vi "Close.vi"(8 "error in (no error)":errorcluster, 11 "SSI PR Settings In":T1={"VISA resource name"="", "Simulated?"=TRUE}) -> (0 "error out":errorcluster, 3 "SSI PR Settings Out":T1={"VISA resource name"="", "Simulated?"=TRUE})   [LabVIEW 2018]
uses:
  SSI PR Settings Cluster.ctl
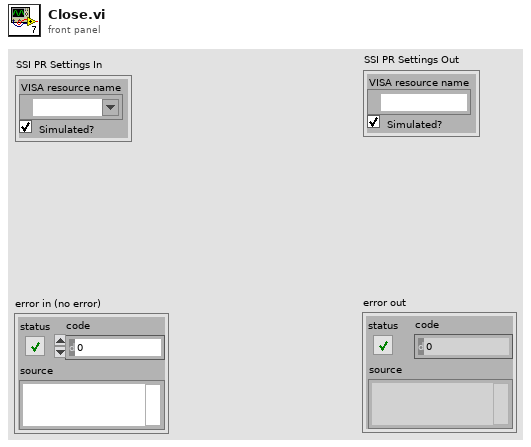
[diagram p1: front panel]
types:
  T1 = typedef "SSI PR Settings Cluster.ctl" = cluster{"VISA resource name":refnum<visa-resource-name>, "Simulated?":bool}
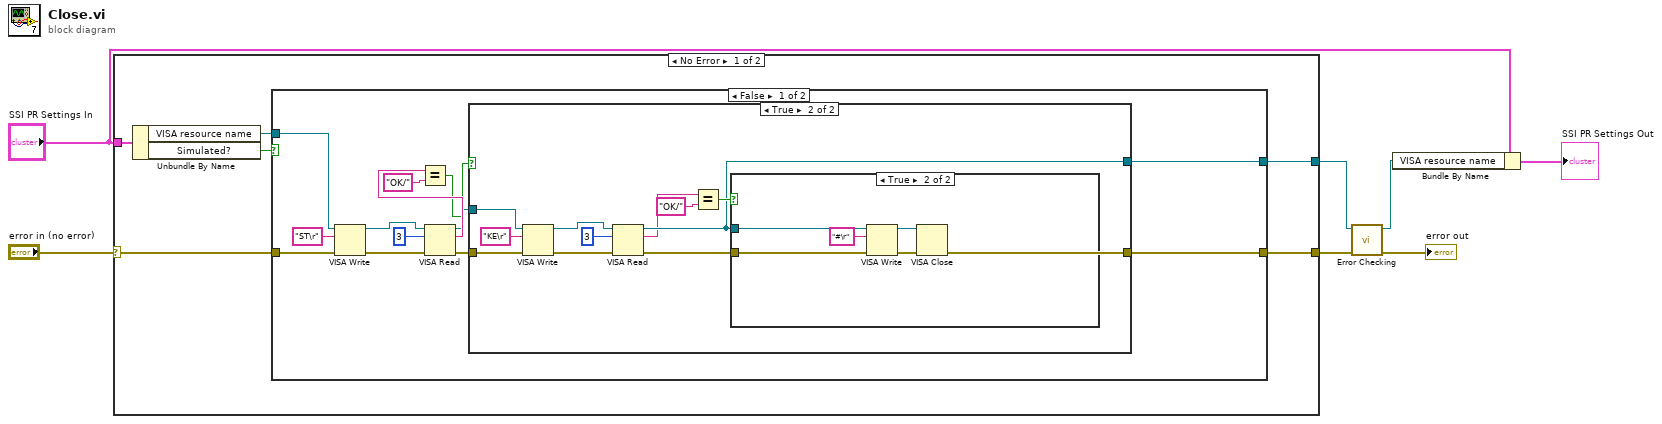
[diagram p0: block diagram]
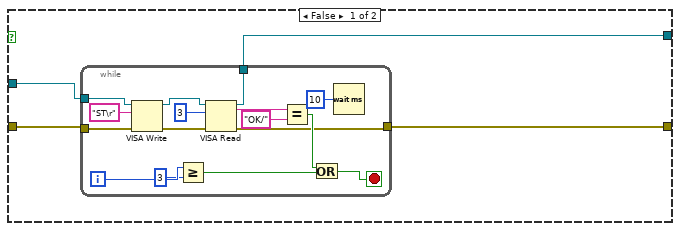
[diagram p2: hidden frame]
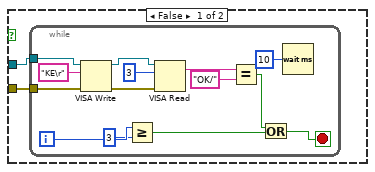
[diagram p3: hidden frame]
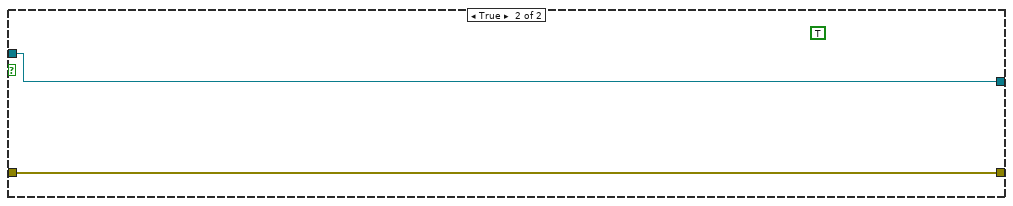
[diagram p4: hidden frame]
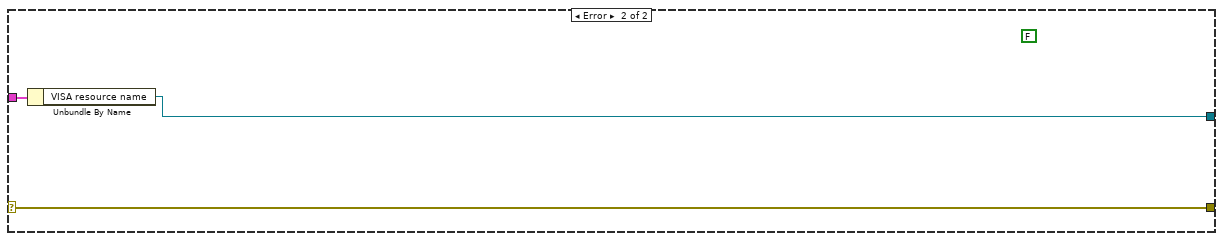
[diagram p5: hidden frame]
diagram:
  n1 = case shown="No Error" "error in (no error)" {
    selector: "error in (no error)" -> [w13 w83]
    tunnel: "SSI PR Settings In" -> [w9 w82]
    tunnel: [w10 w83] -> w4
    tunnel: [w8 w81] -> w3
    frame No Error {
      n2 = Unbundle By Name(w9) -> ("VISA resource name"=w11:refnum<visa-resource-name>, "Simulated?"=w12:bool)
      n3 = case shown="False" w12 {
        tunnel: w13 -> [w20 w80]
        tunnel: w11 -> [w15 w79]
        tunnel: [w26 w80] -> w10
        tunnel: [w25 w79] -> w8
        frame False {
          n4 = VISA Write(VISA resource name=w15, write buffer="ST\r", error in (no error)=w20) -> (VISA resource name out=w22:refnum<visa-resource-name>, error out=w21:errorcluster)  [unwired: 1 out]
          n5 = VISA Read(VISA resource name=w22, byte count=u32 3, error in (no error)=w21) -> (VISA resource name out=w14:refnum<visa-resource-name>, read buffer=w17:string, error out=w19:errorcluster)  [unwired: 1 out]
          n6 = Equal?(x=w17, y="OK/") -> (x = y?=w16:bool)
          n7 = case shown="True" w16 {
            tunnel: w14 -> [w30 w47]
            tunnel: [w28 w54] -> w26
            tunnel: [w27 w53] -> w25
            tunnel: w19 -> [w29 w48]
            frame False {
              n8 = while {
                tunnel: w30 -> [w45]
                tunnel: w29 -> [w44]
                tunnel: [w32] -> w28
                tunnel: [w31] -> w27
                i -> [w36]
                stop <- w37 stop-if-true
                n9 = VISA Write(VISA resource name=w45, write buffer="ST\r", error in (no error)=w44) -> (VISA resource name out=w42:refnum<visa-resource-name>, error out=w41:errorcluster)  [unwired: 1 out]
                n10 = Greater Or Equal?(x=w36, y=3) -> (x >= y?=w34:bool)
                n11 = VISA Read(VISA resource name=w42, byte count=u32 3, error in (no error)=w41) -> (VISA resource name out=w31:refnum<visa-resource-name>, read buffer=w40:string, error out=w32:errorcluster)  [unwired: 1 out]
                n12 = Equal?(x=w40, y="OK/") -> (x = y?=w38:bool)
                n13 = Or(x=w38, y=w34) -> (x .or. y?=w37:bool)
                n14 = Wait (ms)(milliseconds to wait=u32 10) -> ()  [unwired: 1 out]
              }
            }
            frame True {
              n15 = VISA Write(VISA resource name=w47, write buffer="KE\r", error in (no error)=w48) -> (VISA resource name out=w50:refnum<visa-resource-name>, error out=w49:errorcluster)  [unwired: 1 out]
              n16 = VISA Read(VISA resource name=w50, byte count=u32 3, error in (no error)=w49) -> (VISA resource name out=w53:refnum<visa-resource-name>, read buffer=w51:string, error out=w54:errorcluster)  [unwired: 1 out]
              n17 = Equal?(x=w51, y="OK/") -> (x = y?=w55:bool)
              n18 = case shown="True" w55 {
                tunnel: w53 -> [w59 w77]
                tunnel: w54 -> [w58 w76]
                frame False {
                  n19 = while {
                    tunnel: w59 -> [w72]
                    tunnel: w58 -> [w71]
                    i -> [w63]
                    stop <- w64 stop-if-true
                    n20 = VISA Write(VISA resource name=w72, write buffer="KE\r", error in (no error)=w71) -> (VISA resource name out=w69:refnum<visa-resource-name>, error out=w68:errorcluster)  [unwired: 1 out]
                    n21 = Greater Or Equal?(x=w63, y=3) -> (x >= y?=w61:bool)
                    n22 = VISA Read(VISA resource name=w69, byte count=u32 3, error in (no error)=w68) -> (read buffer=w67:string)  [unwired: 3 out]
                    n23 = Equal?(x=w67, y="OK/") -> (x = y?=w65:bool)
                    n24 = Or(x=w65, y=w61) -> (x .or. y?=w64:bool)
                    n25 = Wait (ms)(milliseconds to wait=u32 10) -> ()  [unwired: 1 out]
                  }
                }
                frame True {
                  n26 = VISA Write(VISA resource name=w77, write buffer="#\r", error in (no error)=w76) -> (VISA resource name out=w75:refnum<visa-resource-name>, error out=w74:errorcluster)  [unwired: 1 out]
                  n27 = VISA Close(VISA resource name=w75, error in (no error)=w74) -> ()  [unwired: 1 out]
                }
              }
            }
          }
        }
        frame True {
          (unwired) TRUE
        }
      }
    }
    frame Error {
      (unwired) FALSE
      n28 = Unbundle By Name(w82) -> ("VISA resource name"=w81:refnum<visa-resource-name>)
    }
  }
  n29 = call "Error Checking.vi"("error in (no error)"=w4, "VISA resource name"=w3) -> ("error out"=→"error out":errorcluster, "VISA resource name"=w6:refnum<visa-resource-name>)  [unwired: 7 in, 1 out]
  n30 = Bundle By Name(cluster="SSI PR Settings In", "VISA resource name"=w6) -> (→"SSI PR Settings Out":T1)
